vi "Set Admin Visible .vi"(8 "error in (no error)":errorcluster, 10 "Visible":bool, 11 "Login Refs":T1) -> (0 "error out":errorcluster)   [LabVIEW 2026]
uses:
  controls/UI/Login Refs.ctl
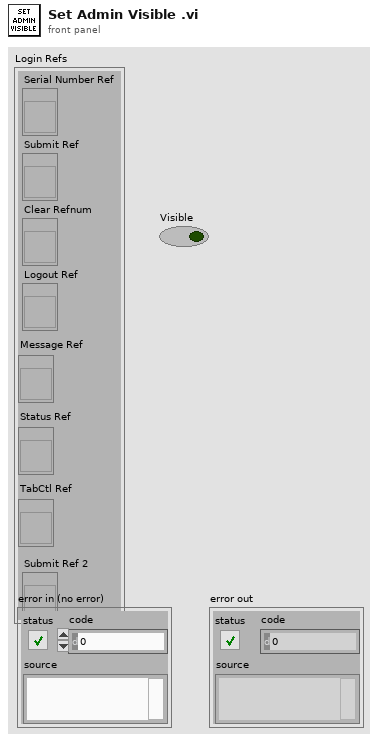
[diagram p1: front panel]
types:
  T1 = typedef "Login Refs.ctl" = cluster{"Serial Number Ref":refnum<vi>, "Submit Ref":refnum<vi>, "Clear Refnum ":refnum<vi>, "Logout Ref":refnum<vi>, "Message Ref":refnum<vi>, "Status Ref":refnum<vi>, "TabCtl Ref":refnum<vi>, "Submit Ref 2":refnum<vi>}
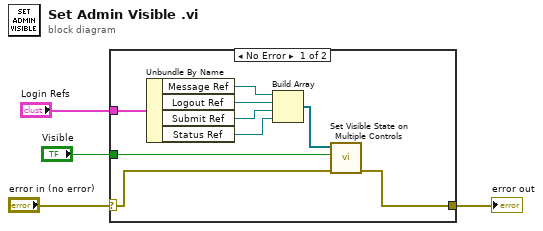
[diagram p0: block diagram]
diagram:
  n1 = case shown="No Error" "error in (no error)" {
    selector: "error in (no error)" -> [w6 w14]
    tunnel: [w13 w14] -> w4
    tunnel: "Login Refs" -> [w12 _]
    tunnel: "Visible" -> [w7 _]
    frame No Error {
      n2 = Unbundle By Name(w12) -> ("Message Ref"=w8:refnum<vi>, "Logout Ref"=w9:refnum<vi>, "Submit Ref"=w10:refnum<vi>, "Status Ref"=w5:refnum<vi>)
      n3 = Build Array(w8, w9, w10, w5) -> (w11:refnum<vi>[])
      n4 = call "Set Visible State on Multiple Controls.vi"("error in (no error)"=w6, "Visible?"=w7, "Controls"=w11) -> ("error out"=w13:errorcluster)  [unwired: 8 in]
    }
    frame Error {
    }
  }
  "error out" <- w4
